vi "remove channel by name.vi"(8 "error in (no error)":errorcluster, 10 "name":string, 11 "E2E configuration in":refnum<class "E2E Tag Exchange configuration.lvclass">) -> (0 "error out":errorcluster, 2 "removed channel":refnum<class "TBM channel.lvclass">, 3 "E2E configuration out":refnum<class "E2E Tag Exchange configuration.lvclass">)   [LabVIEW 2015, in "E2E Tag Exchange configuration.lvclass"]
uses:
  E2E Tag Exchange configuration.lvclass
  <vilib>/NI/Tag Bus Module Framework/channel/TBM channel.lvclass
  E2E Tag Exchange configuration.lvclass/E2E Tag Exchange configuration.ctl
  <vilib>/NI/Tag Bus/tag/tag descriptor.lvclass/tag descriptor.ctl
  <vilib>/NI/Tag Bus/tag/read tag name.vi
  <vilib>/NI/Tag Bus/tag/tag descriptor.lvclass
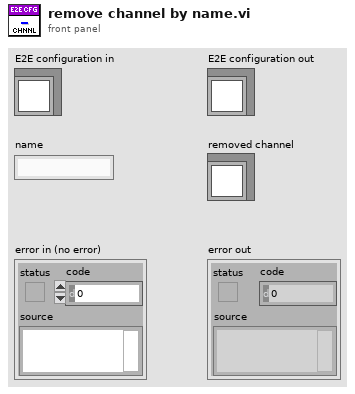
[diagram p1: front panel]
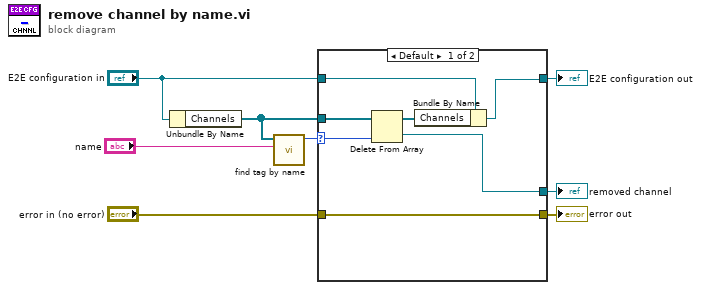
[diagram p0: block diagram]
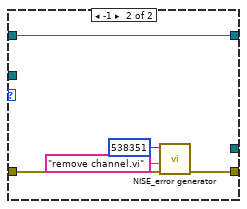
[diagram p2: hidden frame]
diagram:
  n1 = Unbundle By Name("E2E configuration in") -> ("Channels"=w6:refnum<class "TBM channel.lvclass">[])
  n2 = call <vilib>:"find tag by name.vi"("name"="name", "tags in"=w6) -> ("index"=w7:i32)  [unwired: 9 in]
  n3 = case shown="Default" w7 {
    selector: w7 -> [w11 _]
    tunnel: "E2E configuration in" -> [w15 w20]
    tunnel: w6 -> [w14 _]
    tunnel: [w9 w19] -> w5
    tunnel: [w13 w20] -> w4
    tunnel: [w10 _] -> w3
    tunnel: "error in (no error)" -> [w9 w16]
    frame Default {
      n4 = Delete From Array(array=w14, index=w11) -> (deleted portion=w10:refnum<class "TBM channel.lvclass">, array with subset deleted=w12:refnum<class "TBM channel.lvclass">[])  [unwired: 1 in]
      n5 = Bundle By Name(cluster=w15, "Channels"=w12) -> (w13:refnum<class "E2E Tag Exchange configuration.lvclass">)
    }
    frame -1 {
      n6 = call <vilib>:"NISE_error generator.vi"("error in"=w16, "source"="remove channel.vi", "error code (0)"=538351) -> ("error out"=w19:errorcluster)  [unwired: 6 in]
    }
  }
  "error out" <- w5
  "E2E configuration out" <- w4
  "removed channel" <- w3
